vi "Write Network Master.vi"(8 "error in":errorcluster, 10 "Network Master":refnum<class "Network Master.lvclass">, 11 "Modbus master in":refnum<class "Modbus Master CR API.lvclass">) -> (0 "error out":errorcluster, 3 "Modbus master out":refnum<class "Modbus Master CR API.lvclass">)   [LabVIEW 2021, in "Modbus Master CR API.lvclass"]
doc: "This VI is an accessor for the function definition stored in the Modbus master instance. This accessor can be used as a property node. This function definition is used by the master to determine how to pack and unpack Modbus protocol data units."
uses:
  Modbus Master CR API.lvclass
  Modbus Master CR API.lvclass/Modbus Master CR API.ctl
  Network Protocol/Network Master/Network Master.lvclass
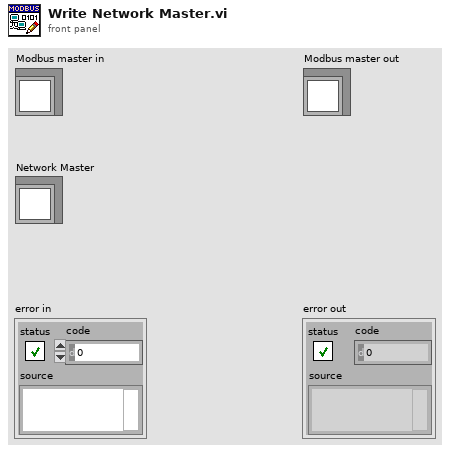
[diagram p1: front panel]
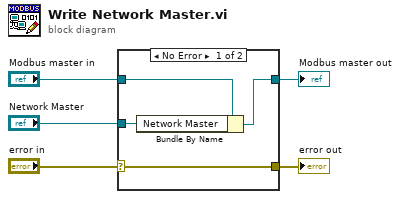
[diagram p0: block diagram]
diagram:
  n1 = case shown="No Error" "error in" {
    selector: "error in" -> [w6 w10]
    tunnel: "Network Master" -> [w9 _]
    tunnel: "Modbus master in" -> [w8 w11]
    tunnel: [w7 w11] -> w3
    tunnel: [w6 w10] -> w1
    frame No Error {
      n2 = Bundle By Name(cluster=w8, "Network Master"=w9) -> (w7:refnum<class "Modbus Master CR API.lvclass">)
    }
    frame Error {
    }
  }
  "error out" <- w1
  "Modbus master out" <- w3
